vi "Header or Footer Create or Modify PdfPTable.vi"(2 "Header or Footer":T11, 7 "pageNum":i32=1, 9 "Header Footer IN [ ]":T1, 11 "error in (no error)":errorcluster, 12 "Page points":T12={"Start at page"=612, "Orientation"=enum."Portrait", "widht"=612.0, "height"=792.0, "Margin left"=70.86614, "Margin right"=70.86614, "Margin top"=70.8661, "Margin bottom"=70.8661}) -> (6 "Modify Image Cell":bool, 10 "Header Footer OUT [ ]":T1, 15 "error out":errorcluster)   [LabVIEW 2013]
doc: "Version 1.0\nDeveloped by Jean-Marc Simard\nCopyright © 2010, Exaprom Inc.\nAll rights reserved.\nLicense: BSD\n\nWith iTextSharp 4.1.6 (http://itextsharp.sourceforge.net)\nunder Mozilla Public License Version 1.1\n(http://www.mozilla.org/MPL/MPL-1.1.html)"
uses:
  Controls/Page dimensions.ctl
  Controls/Page Orientation.ctl
  Controls/Header or Footer.ctl
  Controls/Header Footer Complete Cluster.ctl
  Controls/Header Footer Cluster with references.ctl
  Controls/Header Footer Type.ctl
  Controls/Header footer horiz alignment.ctl
  Controls/Cell Vertical alignment.ctl
  Controls/Page number.ctl
  C:/Users/MaxCorp/Documents/GitHub/TopView/DLL/itextsharp.dll
  DLL/itextsharp.dll
  Controls/Font cluster.ctl
  Controls/Font size.ctl
  Controls/Font color.ctl
  Controls/Header Footer Line.ctl
  Controls/Table position.ctl
panel:
  # "X"
  # "Y"
  # "X"
  # "Y"
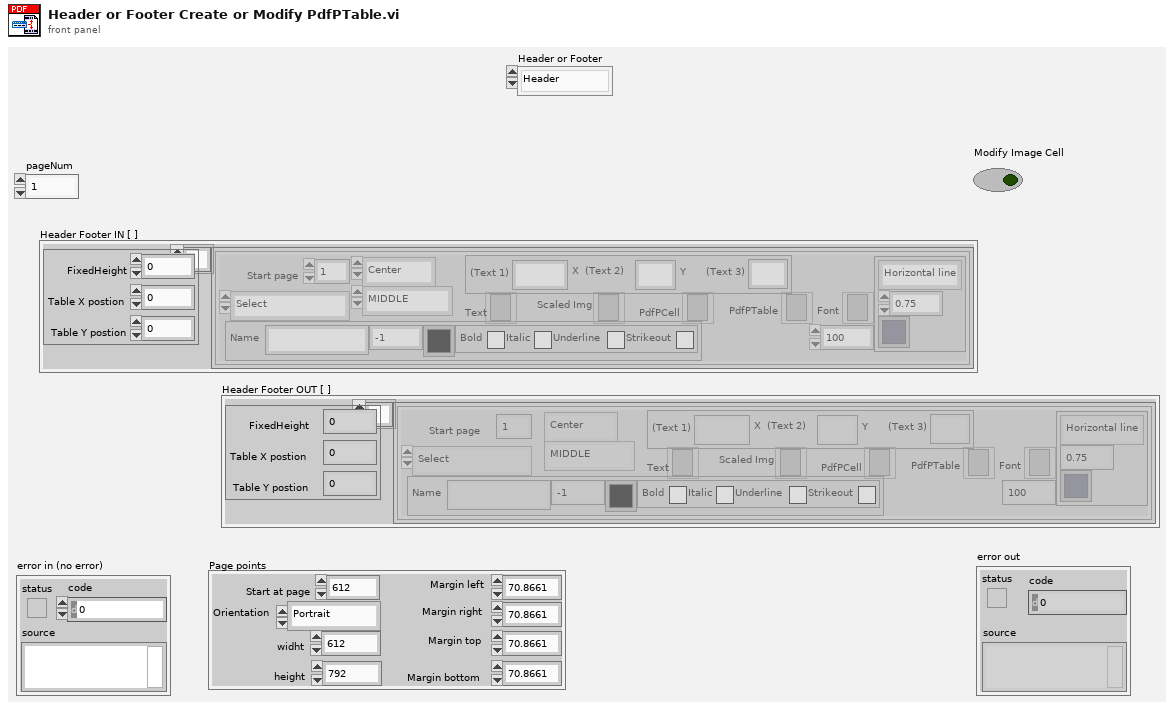
[diagram p1: front panel]
types:
  T1 = typedef "Header Footer Complete Cluster.ctl" = cluster{"Table position":cluster{"FixedHeight":dbl, "Table X postion":dbl, "Table Y postion":dbl}, "Header Footer Cluster with references [ ]":T2[]}
  T2 = typedef "Header Footer Cluster with references.ctl" = cluster{"Start page":i32, "Type":T3, "Alignment":T4, "Vertical Alignement":T5, "Page #":T6, "Text":refnum<k24>, "Scaled Img":refnum<k24>, "PdfPCell":refnum<k24>, "PdfPTable":refnum<k24>, "Font Cluster":T7, "Font ":refnum<k24>, "Img (%)":sgl, "Line":cluster{"Line":T10, "Thickness (points)":sgl, "Colour":T9}}
  T3 = typedef "Header Footer Type.ctl" = enum16{"Select", "Text", "Text + hyperlink", "Page number", "Image", "Image + hyperlink"}
  T4 = typedef "Header footer horiz alignment.ctl" = enum16{"Left", "Center", "Right"}
  T5 = typedef "Cell Vertical alignment.ctl" = enum16{"TOP", "MIDDLE", "BOTTOM"}
  T6 = typedef "Page number.ctl" = cluster{"Text 1":string, "Text 2":string, "Text 3":string}
  T7 = typedef "Font cluster.ctl" = cluster{"Name":string, "Size":T8, "Color":T9, "Style":cluster{"Bold":bool, "Italic":bool, "Underline":bool, "Strikeout":bool}}
  T8 = typedef "Font size.ctl" = sgl
  T9 = typedef "Font color.ctl" = u32
  T10 = typedef "Header Footer Line.ctl" = enum16{"No line", "Horizontal line"}
  T11 = typedef "Header or Footer.ctl" = enum16{"Header", "Footer"}
  T12 = typedef "Page dimensions.ctl" = cluster{"Start at page":i32, "Orientation":T13, "widht":sgl, "height":sgl, "Margin left":sgl, "Margin right":sgl, "Margin top":sgl, "Margin bottom":sgl}
  T13 = typedef "Page Orientation.ctl" = enum16{"Portrait", "Landscape"}
  T14 = cluster{"FixedHeight":dbl, "Table X postion":dbl, "Table Y postion":dbl}
  T15 = typedef "Table position.ctl" = i32
  T16 = cluster{"Table position":cluster{"FixedHeight":dbl, "Table X postion":dbl, "Table Y postion":dbl}, "Header Footer Cluster with references [ ]":T2[]}
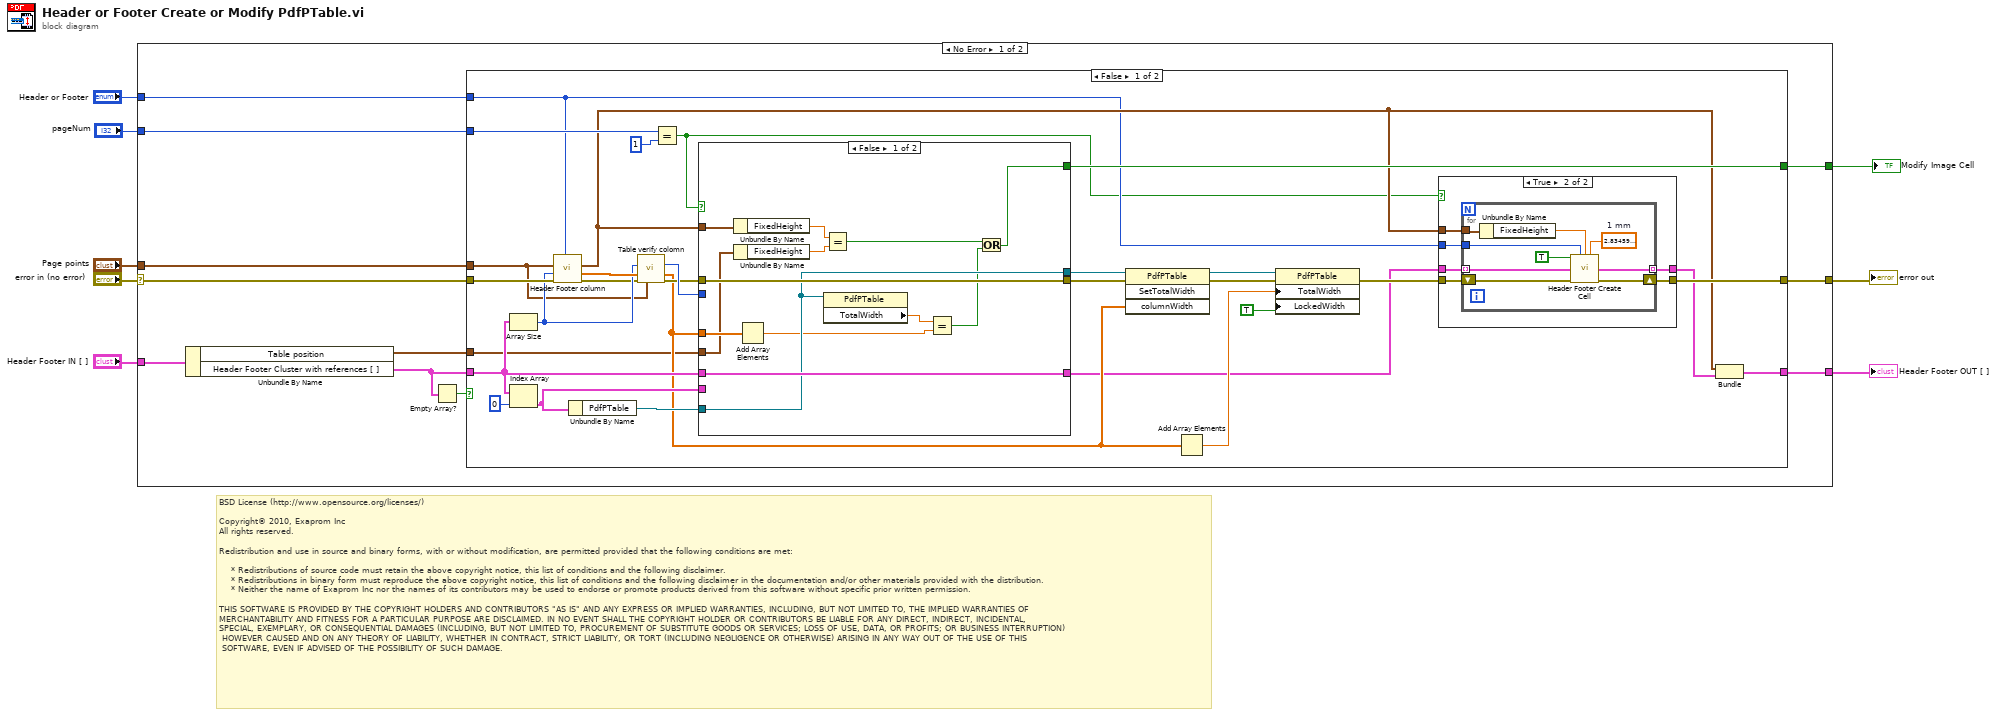
[diagram p0: block diagram]
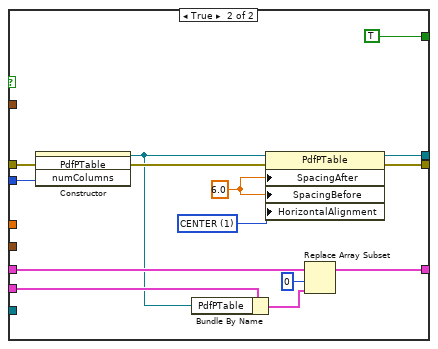
[diagram p3: hidden frame]
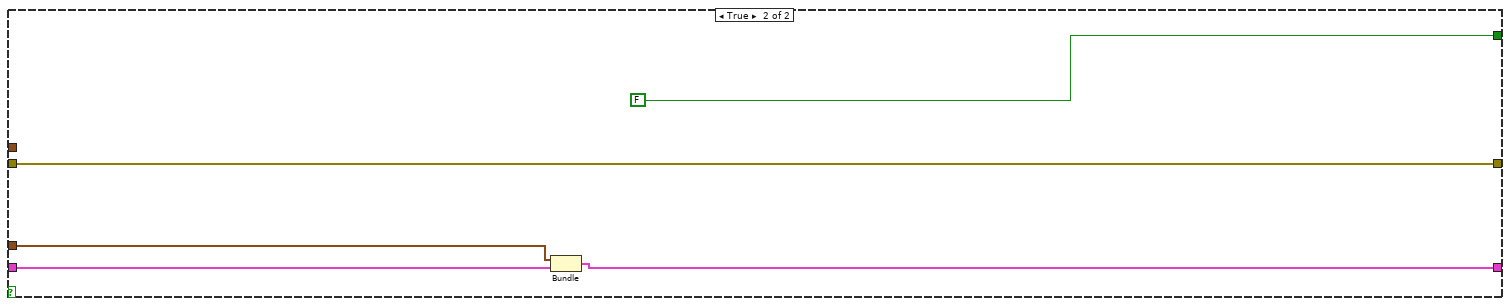
[diagram p4: hidden frame]
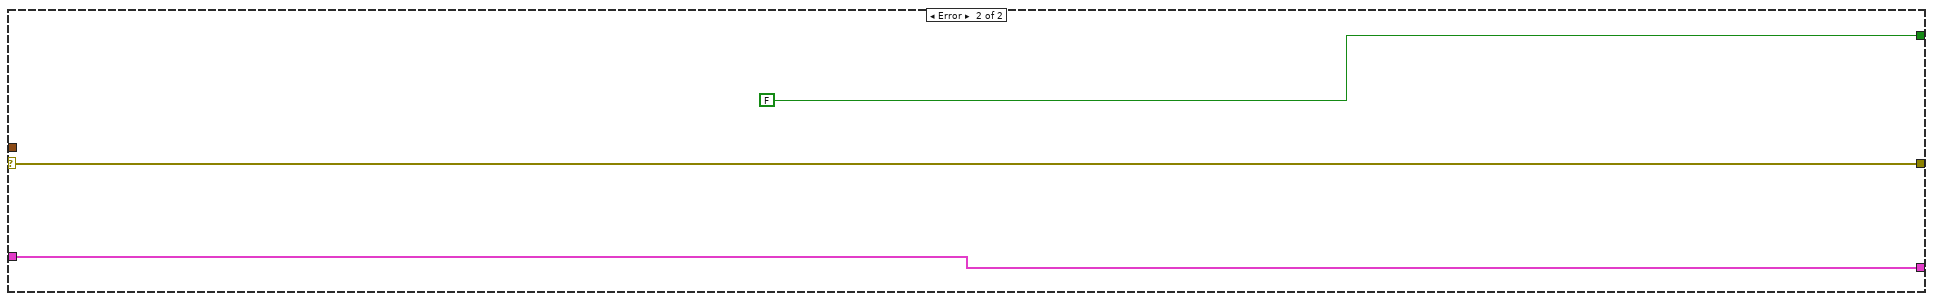
[diagram p5: hidden frame]
diagram:
  # "BSD License (http://www.opensource.org/licenses/)\n\nCopyright© 2010, Exaprom Inc\nAll rights reserved.\n\nRedistribution and use in source and binary forms, with or without modification, are permitted provided that the following conditions are met:\n\n    * Redistributions of source code must retain the above copyright notice, this list of conditions and the following disclaimer.\n    * Redistributions in binary form must reproduce the above copyright notice, this list of conditions and the following disclaimer in the documentation and/or other materials provided with the distribution.\n    * Neither the name of Exaprom Inc nor the names of its contributors may be used to endorse or promote products derived from this software without specific prior written permission.\n\nTHIS SOFTWARE IS PROVIDED BY THE COPYRIGHT HOLDERS AND CONTRIBUTORS \"AS IS\" AND ANY EXPRESS OR IMPLIED WARRANTIES, INCLUDING, BUT NOT LIMITED TO, THE IMPLIED WARRANTIES OF \nMERCHANTABILITY AND FITNESS FOR A PARTICULAR PURPOSE ARE DISCLAIMED. IN NO EVENT SHALL THE COPYRIGHT HOLDER OR CONTRIBUTORS BE LIABLE FOR ANY DIRECT, INDIRECT, INCIDENTAL,\nSPECIAL, EXEMPLARY, OR CONSEQUENTIAL DAMAGES (INCLUDING, BUT NOT LIMITED TO, PROCUREMENT OF SUBSTITUTE GOODS OR SERVICES; LOSS OF USE, DATA, OR PROFITS; OR BUSINESS INTERRUPTION)\n HOWEVER CAUSED AND ON ANY THEORY OF LIABILITY, WHETHER IN CONTRACT, STRICT LIABILITY, OR TORT (INCLUDING NEGLIGENCE OR OTHERWISE) ARISING IN ANY WAY OUT OF THE USE OF THIS\n SOFTWARE, EVEN IF ADVISED OF THE POSSIBILITY OF SUCH DAMAGE."
  n1 = case shown="No Error" "error in (no error)" {
    selector: "error in (no error)" -> [w16 w101]
    tunnel: [w18 w101] -> w8
    tunnel: "pageNum" -> [w19 _]
    tunnel: "Page points" -> [w17 _]
    tunnel: "Header or Footer" -> [w15 _]
    tunnel: "Header Footer IN [ ]" -> [w13 w100]
    tunnel: [w9 w100] -> w2
    tunnel: [w11 FALSE] -> w1
    frame No Error {
      n2 = Unbundle By Name(w13) -> ("Table position"=w10:T14, "Header Footer Cluster with references [ ]"=w12:T2[])
      n3 = Empty Array?(array=w12) -> (empty?=w14:bool)
      n4 = case shown="False" w14 {
        tunnel: w19 -> [w36 _]
        tunnel: [w28 w98] -> w18
        tunnel: w17 -> [w39 _]
        tunnel: w16 -> [w49 w98]
        tunnel: w15 -> [w22 _]
        tunnel: [w25 w94] -> w9
        tunnel: w12 -> [w31 w96]
        tunnel: [w26 FALSE] -> w11
        tunnel: w10 -> [w29 w95]
        frame False {
          n5 = Array Size(array=w31) -> (size(s)=w41:i32)
          n6 = Index Array(array=w31, index=0) -> (element=w32:T2)
          n7 = call "Header Footer column.vi"("Header or Footer"=w22, "error in (no error)"=w49, "numColumns"=w41, "Page points"=w39) -> ("error out"=w40:errorcluster, "Table Column"=w42:dbl[], "Table position"=w23:T14)  [unwired: 5 out]
          n8 = Unbundle By Name(w32) -> ("PdfPTable"=w33:refnum<k24>)
          n9 = call "Table verify colomn.vi"("numColumns"=w41, "columnWidth"=w42, "error in (no error)"=w40, "Pages dimensions"=w39) -> ("numColumns duplicate"=w48:i32, "columnWidth (points)"=w30:sgl[], "error out"=w47:errorcluster)  [unwired: 1 in, 8 out]
          n10 = Equal?(x=w36, y=1) -> (x = y?=w21:bool)
          n11 = case shown="False" w21 {
            tunnel: w48 -> [_ w93]
            tunnel: w47 -> [w79 w92]
            tunnel: [w79 w89] -> w38
            tunnel: [w77 w88] -> w37
            tunnel: w33 -> [w77 _]
            tunnel: w31 -> [w78 w86]
            tunnel: w32 -> [_ w85]
            tunnel: [w78 w81] -> w24
            tunnel: [w68 TRUE] -> w26
            tunnel: w23 -> [w73 _]
            tunnel: w30 -> [w76 _]
            tunnel: w29 -> [w72 _]
            frame False {
              n12 = Unbundle By Name(w73) -> ("FixedHeight"=w71:dbl)
              n13 = Unbundle By Name(w72) -> ("FixedHeight"=w70:dbl)
              n14 = Add Array Elements(numeric array=w76) -> (sum=w74:sgl)
              n15 = property class="PdfPTable"(reference=w77) -> ("TotalWidth"=w75:sgl)  [unwired: 1 in, 2 out]
              n16 = Equal?(x=w71, y=w70) -> (x = y?=w67:bool)
              n17 = Equal?(x=w75, y=w74) -> (x = y?=w69:bool)
              n18 = Or(x=w67, y=w69) -> (x .or. y?=w68:bool)
            }
            frame True {
              w87 = T15 1 items=["LEFT", "CENTER", "RIGHT"] ("Table position")
              w91 = sgl 6.0 ("SpacingAfter")
              n19 = constructor class="PdfPTable"(error in=w92, "numColumns"=w93) -> (reference out=w84:refnum<k24>, error out=w90:errorcluster)  [unwired: 2 in, 2 out]
              n20 = Bundle By Name(cluster=w85, "PdfPTable"=w84) -> (w83:T2)
              n21 = property class="PdfPTable"(reference=w84, error in=w90, "SpacingAfter"=w91, "SpacingBefore"=w91, "HorizontalAlignment"=w87) -> (reference out=w88:refnum<k24>, error out=w89:errorcluster)
              n22 = Replace Array Subset(array=w86, new element=w83, index=0) -> (w81:T2[])
            }
          }
          n23 = invoke class="PdfPTable" method="SetTotalWidth"(reference=w37, error in=w38, "columnWidth"=w30) -> (reference out=w43:refnum<k24>, error out=w44:errorcluster)  [unwired: 1 in, 2 out]
          n24 = Add Array Elements(numeric array=w30) -> (sum=w46:sgl)
          n25 = property class="PdfPTable"(reference=w43, error in=w44, "TotalWidth"=w46, "LockedWidth"=TRUE) -> (error out=w27:errorcluster)  [unwired: 1 out]
          n26 = case shown="True" w21 {
            tunnel: [w51 w57] -> w28
            tunnel: w27 -> [w51 w56]
            tunnel: w24 -> [w50 w55]
            tunnel: w23 -> [_ w54]
            tunnel: w22 -> [_ w53]
            tunnel: [w50 w52] -> w20
            frame False {
            }
            frame True {
              n27 = for {
                shift-right: [w64] -> w57
                shift-left: w56 -> [w63]
                tunnel: w55 -> [w62] mode=indexing
                tunnel: w54 -> [w61]
                tunnel: w53 -> [w59]
                tunnel: [w58] -> w52 mode=indexing
                w65 = sgl 2.8346  # 1 mm
                n28 = Unbundle By Name(w61) -> ("FixedHeight"=w60:dbl)
                n29 = call "Header Footer Create Cell.vi"("Change format?"=TRUE, "Header or Footer"=w59, "FixedHeight (points)"=w60, "Padding (points)"=w65, "Header Footer Cluster with references IN"=w62, "error in (no error)"=w63) -> ("Header Footer Cluster with references OUT"=w58:T2, "error out"=w64:errorcluster)  [unwired: 2 in, 6 out]
              }
            }
          }
          n30 = Bundle("Table position"=w23, "Header Footer Cluster with references [ ]"=w20) -> (w25:T16)  [unwired: 1 out]
        }
        frame True {
          n31 = Bundle("Table position"=w95, "Header Footer Cluster with references [ ]"=w96) -> (w94:T16)  [unwired: 1 out]
        }
      }
    }
    frame Error {
    }
  }
  "error out" <- w8
  "Header Footer OUT [ ]" <- w2
  "Modify Image Cell" <- w1
